vi "Finalize.vi"(8 "error in":errorcluster, 11 "Plugin in":refnum<class "StreamReader.lvclass">) -> (0 "error out":errorcluster, 3 "Plugin out":refnum<class "StreamReader.lvclass">)   [LabVIEW 2024, in "StreamReader.lvlib" / "StreamReader.lvclass"]
uses:
  StreamReader.lvclass
  StreamReader.lvclass/StreamReader.ctl
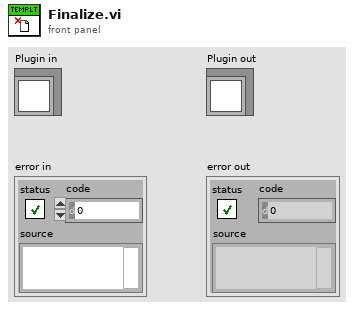
[diagram p1: front panel]
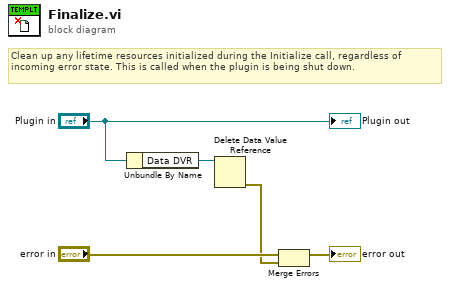
[diagram p0: block diagram]
diagram:
  # "Clean up any lifetime resources initialized during the Initialize call, regardless of incoming error state. This is called when the plugin is being shut down."
  n1 = Unbundle By Name("Plugin in") -> ("Data DVR"=w2:refnum<data-value>)
  n2 = Delete Data Value Reference(data value reference=w2) -> (error out=w1:errorcluster)  [unwired: 1 in, 1 out]
  n3 = Merge Errors("error in", w1) -> (→"error out":errorcluster)
  "Plugin out" <- "Plugin in"
